vi "merge tdms files.vi"(0 "save to":path, 5 "merge paths":path[](array[path])) -> (14 "Dateipfad (Ausgang)":path, 19 "Fehler (Ausgang)":errorcluster)   [LabVIEW 2017, in "util.lvlib"]
uses:
  util.lvlib
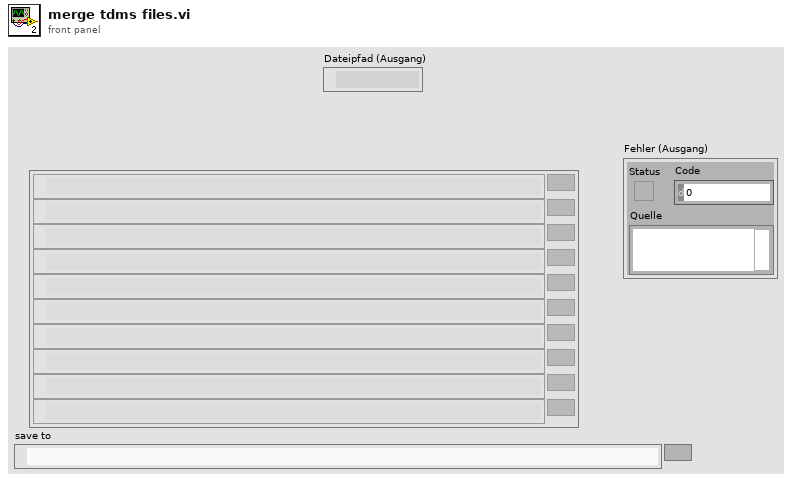
[diagram p1: front panel]
types:
  T1 = enum16{"open", "open or create", "create or replace", "create", "open (read-only)"}
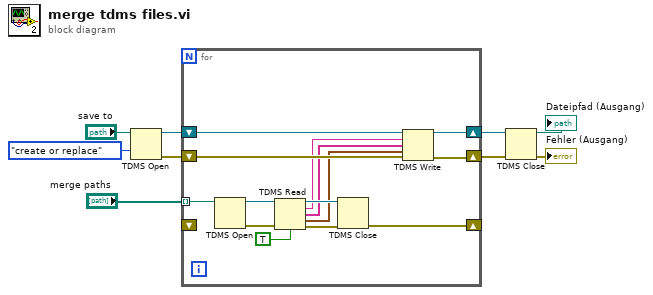
[diagram p0: block diagram]
diagram:
  n1 = TDMS Open(10:T1."create or replace" ("Operation (0:Öffnen)"), 11:"save to") -> (0:w8:errorcluster, 3:w9:refnum<k34>)  [unwired: 5 in]
  n2 = for {
    tunnel: "merge paths" -> [w23] mode=indexing
    shift-right: [w18] -> _
    shift-left: _ -> [_]
    shift-right: [w14] -> w7
    shift-left: w8 -> [w15]
    shift-right: [w16] -> w6
    shift-left: w9 -> [w17]
    n3 = TDMS Open(11:w23) -> (0:w20:errorcluster, 3:w22:refnum<k34>)  [unwired: 6 in]
    n4 = TDMS Read(0:w22, 11:w20, 13:TRUE ("Kanalreihenfolge von Datei beibehalten? (F)")) -> (4:w21:refnum<k34>, 6:w13:string, 8:w12:string[], 10:w11:waveform(dbl)[], 15:w19:errorcluster)  [unwired: 5 in, 1 out]
    n5 = TDMS Close(8:w19, 11:w21) -> (0:w18:errorcluster)  [unwired: 1 out]
    n6 = TDMS Write(0:w17, 5:w13, 7:w12, 9:w11, 11:w15) -> (4:w16:refnum<k34>, 15:w14:errorcluster)  [unwired: 1 in, 2 out]
  }
  n7 = TDMS Close(8:w7, 11:w6) -> (0:→"Fehler (Ausgang)":errorcluster, 3:→"Dateipfad (Ausgang)":path)
